vi "Event Text For Unregister Many.vi"(10 "guest":string, 11 "strings":string[](array[string])) -> (3 "string":string)   [LabVIEW 2023]
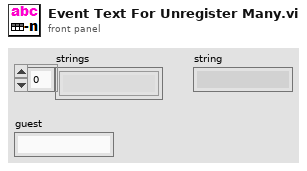
[diagram p1: front panel]
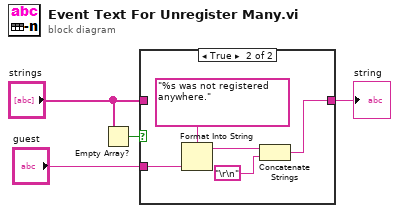
[diagram p0: block diagram]
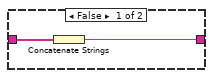
[diagram p2: hidden frame]
diagram:
  n1 = Empty Array?(array="strings") -> (empty?=w3:bool)
  n2 = case shown="True" w3 {
    tunnel: "strings" -> [w6 _]
    tunnel: [w5 w8] -> w1
    tunnel: "guest" -> [_ w10]
    frame False {
      n3 = Concatenate Strings(w6) -> (w5:string)
    }
    frame True {
      n4 = Format Into String(format string="%s was not registered anywhere." ("L10n_message"), w10) -> (resulting string=w9:string)  [unwired: 2 in, 1 out]
      n5 = Concatenate Strings(w9, "\r\n") -> (w8:string)
    }
  }
  "string" <- w1
